vi "CRYProbe Window Check .vi"(10 "Row":i32, 11 "Probe Type":string) -> (2 "Probe VI Ref":refnum<vi>, 3 "Exist?":bool)   [LabVIEW 2013]
uses:
  Global/CRYCurve Library Global.vi
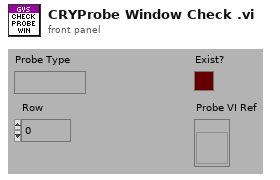
[diagram p1: front panel]
types:
  T1 = typedef "CRYData Cluster.ctl" = cluster{"Name":string, "Curve":cluster{"x":dbl, "y":dbl, "z":dbl}[], "X data":u16, "Y data":u16, "Z data":u16, "X axis":u16, "Y axis":u16, "Z axis":u16, "X unit":string, "Y unit":string, "Z unit":string, "X dB ref":dbl, "Y dB ref":dbl, "Z dB ref":dbl, "single val":bool, "protected":bool, "display X":bool, "display Y":bool, "display Z":bool, "Test Info":string, "Step No.":i32, "Plot Settings":cluster{"Color":u32, "Interpolation":u8, "Point Style":u8, "Line Style":u8, "Point Color":u32, "Line Width":u8, "Bar Plot Style":u8, "Fill To":i16}, "AutoProtect":bool}
  T2 = typedef "CRYWaveform Cluster.ctl" = cluster{"Waveform":cluster{"X0":dbl, "dX":dbl, "Y":sgl[]}, "X data":u16, "Y data":u16, "Y axis":u16, "X unit":string, "Y unit":string, "Y dB ref":dbl, "display Y":bool, "display X":bool, "Overload?":bool, "Test Info":string, "Step No.":i32, "Name":string, "protected":bool, "Sqc history":string[], "Signal Channel ID":i32, "Plot Settings":cluster{"Color":u32, "Interpolation":u8, "Point Style":u8, "Line Style":u8, "Point Color":u32, "Line Width":u8, "Bar Plot Style":u8, "Fill To":i16}, "AutoProtect":bool}
  T3 = typedef "CRYResult Cluster.ctl" = cluster{"Name":string, "Margin":dbl, "unit":string, "Verdict":bool, "Limit":string, "Max/Min":string, "protected":bool, "Step No.":i32, "Test Info":string, "AutoProtect":bool}
  T4 = cluster{"Type Name":string, "Data Name":string, "Probe VIRef Number":i32, "Probe VIRef":refnum<vi>}[]
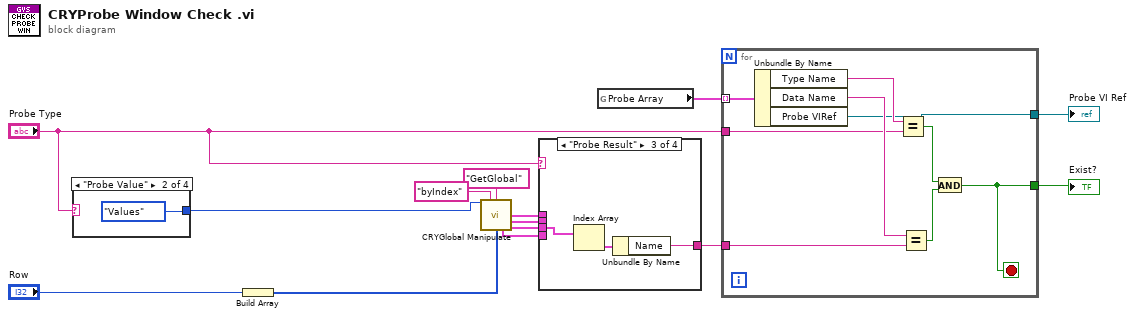
[diagram p0: block diagram]
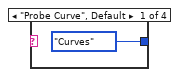
[diagram p2: hidden frame]
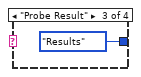
[diagram p3: hidden frame]
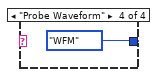
[diagram p4: hidden frame]
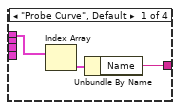
[diagram p5: hidden frame]
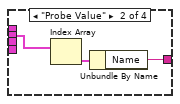
[diagram p6: hidden frame]
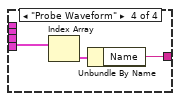
[diagram p7: hidden frame]
diagram:
  n1 = case shown="\"Probe Value\"" "Probe Type" {
    tunnel: [enum16{"Curves", "Values", "Results", "WFM"}."Curves" ("Type") enum16{"Curves", "Values", "Results", "WFM"}."Values" ("Type") enum16{"Curves", "Values", "Results", "WFM"}."Results" ("Type") enum16{"Curves", "Values", "Results", "WFM"}."WFM" ("Type")] -> w2
    frame "Probe Curve", Default {
    }
    frame "Probe Value" {
    }
    frame "Probe Result" {
    }
    frame "Probe Waveform" {
    }
  }
  n2 = Build Array("Row") -> (w1:i32[])
  n3 = call "CRYGlobal Manipulate.vi"("Type"=w2, "sOption"="byIndex", "sAction"="GetGlobal", "nData"=w1) -> ("Curves Out"=w7:T1[], "Values Out"=w6:T1[], "WFM Out"=w4:T2[], "Results Out"=w5:T3[])  [unwired: 5 in, 3 out]
  n4 = case shown="\"Probe Result\"" "Probe Type" {
    tunnel: [w20 w23 w26 w29] -> w14
    tunnel: w7 -> [w19 _ _ _]
    tunnel: w6 -> [_ w22 _ _]
    tunnel: w5 -> [_ _ w25 _]
    tunnel: w4 -> [_ _ _ w28]
    frame "Probe Curve", Default {
      n5 = Index Array(array=w19) -> (element=w21:T1)  [unwired: 1 in]
      n6 = Unbundle By Name(w21) -> ("Name"=w20:string)
    }
    frame "Probe Value" {
      n7 = Index Array(array=w22) -> (element=w24:T1)  [unwired: 1 in]
      n8 = Unbundle By Name(w24) -> ("Name"=w23:string)
    }
    frame "Probe Result" {
      n9 = Index Array(array=w25) -> (element=w27:T3)  [unwired: 1 in]
      n10 = Unbundle By Name(w27) -> ("Name"=w26:string)
    }
    frame "Probe Waveform" {
      n11 = Index Array(array=w28) -> (element=w30:T2)  [unwired: 1 in]
      n12 = Unbundle By Name(w30) -> ("Name"=w29:string)
    }
  }
  n13 = global read "CRYCurve Library Global.vi" "Probe Array"() -> (w11:T4)
  n14 = for {
    tunnel: w11 -> [w39] mode=indexing
    tunnel: w14 -> [w35]
    tunnel: "Probe Type" -> [w36]
    tunnel: [w32] -> w13
    tunnel: [w31] -> w12
    stop <- w32 stop-if-true
    n15 = Unbundle By Name(w39) -> ("Type Name"=w38:string, "Data Name"=w37:string, "Probe VIRef"=w31:refnum<vi>)
    n16 = Equal?(x=w38, y=w36) -> (x = y?=w33:bool)
    n17 = Equal?(x=w37, y=w35) -> (x = y?=w34:bool)
    n18 = And(x=w33, y=w34) -> (x .and. y?=w32:bool)
  }
  "Exist?" <- w13
  "Probe VI Ref" <- w12
